vi "open variable connections.vi"(8 "error in":errorcluster, 11 "variables in":T1[](array[typedef])) -> (0 "error out":errorcluster, 3 "variables out":T1[](array[typedef]))   [LabVIEW 2014, in "Scan Engine runtime.lvclass"]
uses:
  Scan Engine runtime.lvclass
  <vilib>/NI/Tag Bus/tag/Data Type.ctl
  <vilib>/NI/Tag Bus/tag/tag descriptor.lvclass
  Custom Ctrls/Index Map.ctl
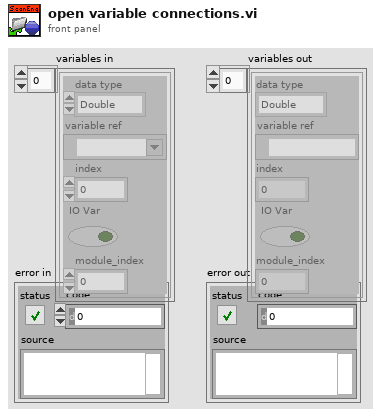
[diagram p1: front panel]
types:
  T1 = typedef "Scan Engine runtime.lvclass/Index Map.ctl" = cluster{"data type":T2, "variable ref":refnum<k21>, "index":i32, "IO Var":bool, "module_index":i32}
  T2 = typedef "tag bus.lvlib/tag descriptor.lvclass/Data Type.ctl" = enum16{"Double", "Single", "I64", "I32", "I16", "I8", "U64", "U32", "U16", "U8", "Boolean", "String", "Array of Double", "Array of Single", "Array of I64", "Array of I32", "Array of I16", "Array of I8", "Array of U64", "Array of U32", "Array of U16", "Array of U8", "Array of Boolean", "Array of String"}
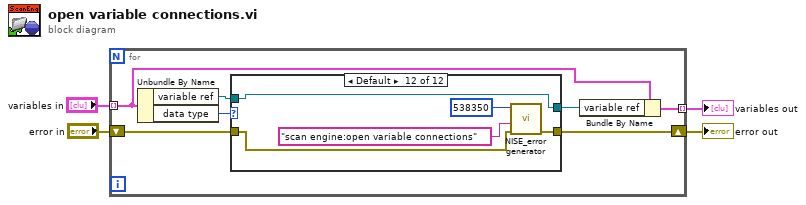
[diagram p0: block diagram]
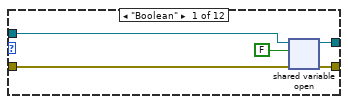
[diagram p2: hidden frame]
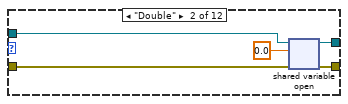
[diagram p3: hidden frame]
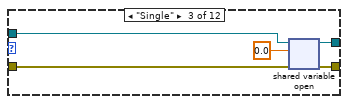
[diagram p4: hidden frame]
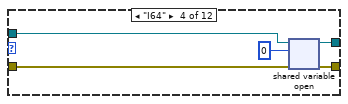
[diagram p5: hidden frame]
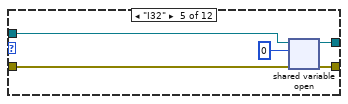
[diagram p6: hidden frame]
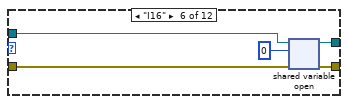
[diagram p7: hidden frame]
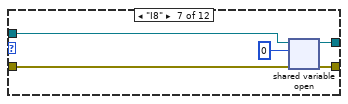
[diagram p8: hidden frame]
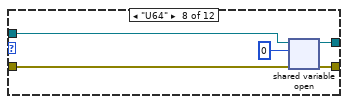
[diagram p9: hidden frame]
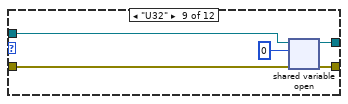
[diagram p10: hidden frame]
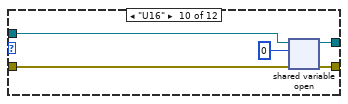
[diagram p11: hidden frame]
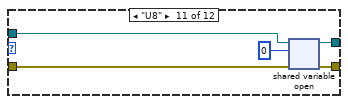
[diagram p12: hidden frame]
diagram:
  n1 = for {
    tunnel: "variables in" -> [w11] mode=indexing
    shift-right: [w6] -> w2
    shift-left: "error in" -> [w5]
    tunnel: [w7] -> w1 mode=indexing
    n2 = Unbundle By Name(w11) -> ("variable ref"=w8:refnum<k21>, "data type"=w10:T2)
    n3 = case shown="Default" w10 {
      tunnel: [w15 w20 w25 w30 w35 w40 w45 w50 w55 w60 w65 w71] -> w9
      tunnel: w8 -> [w16 w21 w26 w31 w36 w41 w46 w51 w56 w61 w66 w71]
      tunnel: [w13 w19 w24 w29 w34 w39 w44 w49 w54 w59 w64 w68] -> w6
      tunnel: w5 -> [w12 w18 w23 w28 w33 w38 w43 w48 w53 w58 w63 w69]
      frame "Boolean" {
        n4 = shared-variable-open(w16, w12, FALSE) -> (w15:refnum<k21>, w13:errorcluster)
      }
      frame "Double" {
        n5 = shared-variable-open(w21, w18, 0.0) -> (w20:refnum<k21>, w19:errorcluster)
      }
      frame "Single" {
        n6 = shared-variable-open(w26, w23, sgl 0.0) -> (w25:refnum<k21>, w24:errorcluster)
      }
      frame "I64" {
        n7 = shared-variable-open(w31, w28, i64 0) -> (w30:refnum<k21>, w29:errorcluster)
      }
      frame "I32" {
        n8 = shared-variable-open(w36, w33, 0) -> (w35:refnum<k21>, w34:errorcluster)
      }
      frame "I16" {
        n9 = shared-variable-open(w41, w38, i16 0) -> (w40:refnum<k21>, w39:errorcluster)
      }
      frame "I8" {
        n10 = shared-variable-open(w46, w43, i8 0) -> (w45:refnum<k21>, w44:errorcluster)
      }
      frame "U64" {
        n11 = shared-variable-open(w51, w48, u64 0) -> (w50:refnum<k21>, w49:errorcluster)
      }
      frame "U32" {
        n12 = shared-variable-open(w56, w53, u32 0) -> (w55:refnum<k21>, w54:errorcluster)
      }
      frame "U16" {
        n13 = shared-variable-open(w61, w58, u16 0) -> (w60:refnum<k21>, w59:errorcluster)
      }
      frame "U8" {
        n14 = shared-variable-open(w66, w63, u8 0) -> (w65:refnum<k21>, w64:errorcluster)
      }
      frame Default {
        n15 = call <vilib>:"NISE_error generator.vi"("error in"=w69, "source"="scan engine:open variable connections", "error code (0)"=538350) -> ("error out"=w68:errorcluster)  [unwired: 6 in]
      }
    }
    n16 = Bundle By Name(cluster=w11, "variable ref"=w9) -> (w7:T1)
  }
  "error out" <- w2
  "variables out" <- w1
